vi "SENS_FOM_RANG_FREQ_DIV.vi"(0 "VISA IN":refnum<visa-resource-name>, 1 "Range number":i32, 2 "Divisor Value":i32, 5 "error in":errorcluster, 7 "Channel":i32) -> (14 "VISA Out":refnum<visa-resource-name>, 19 "error out":errorcluster)   [LabVIEW 2018, in "PNA-X.lvlib"]
doc: "SENSe<cnum>:FOM:RANGe<n>:FREQuency:DIVisor <num> \n(Read-Write) Sets and returns the divisor value. \nThis setting is valid only if the specified range is coupled to the primary range. \nParameters \n<cnum> Any existing channel number; if unspecified, value is set to 1. \n<n> Range number. If unspecified, value is set to 1. \n<num> Divisor value (unitless). \nExamples SENS:FOM:RANG:FREQ:DIV 3 \nsense2:fom:range2:frequency:divisor 0 \nQuery Syntax SENSe<cnum>:FOM:RANGe<n>:FREQuency:DIVisor? \nReturn Type Numeric \nDefault 1 \n1739"
uses:
  PNA-X.lvlib
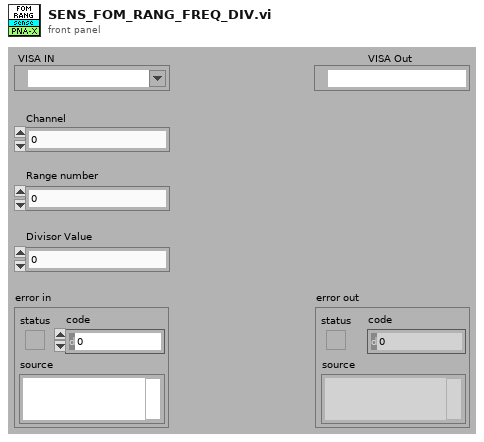
[diagram p1: front panel]
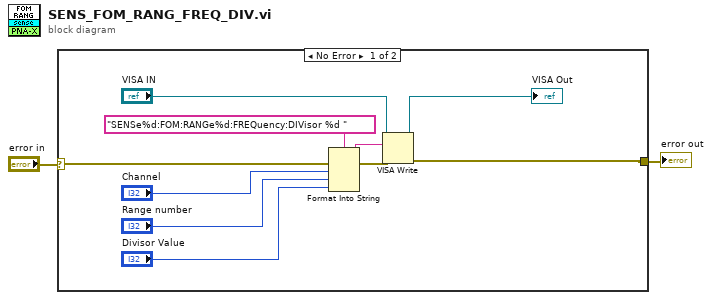
[diagram p0: block diagram]
diagram:
  n1 = case shown="No Error" "error in" {
    selector: "error in" -> [w12 w13]
    tunnel: [w7 w13] -> w1
    frame No Error {
      n2 = Format Into String(format string="SENSe%d:FOM:RANGe%d:FREQuency:DIVisor %d " ("Cmdline"), error in=w12, "Channel", "Range number", "Divisor Value") -> (resulting string=w10:string, error out=w11:errorcluster)  [unwired: 1 in]
      n3 = VISA Write(VISA resource name="VISA IN", write buffer=w10, error in (no error)=w11) -> (VISA resource name out=→"VISA Out":refnum<visa-resource-name>, error out=w7:errorcluster)  [unwired: 1 out]
    }
    frame Error {
    }
  }
  "error out" <- w1
